vi "Initialize RF Sessions From Pinmap.vi"(0 "TSM Context":T1, 11 "error in":errorcluster) -> (4 "RF SubSystem Session Providers":refnum<class "RF Subsystem Session Provider.lvclass">[](array[class]), 15 "error out":errorcluster)   [LabVIEW 2023, in "RFFixtureCharact.Public.lvlib"]
uses:
  RFFixtureCharact.Public.lvlib
  <vilib>/NI_TestStand_SemiconductorModule/NI_TestStand_Semiconductor_Module.lvlibp/PinMap/General/SemiconductorModuleContext.ctl
  Common/RF Subsystem Session Provider/RF Subsystem Session Provider.lvclass
  Common/RFCalAndFixtureCharact.Common.lvlib
  <vilib>/NI_TestStand_SemiconductorModule/NI_TestStand_Semiconductor_Module.lvlibp
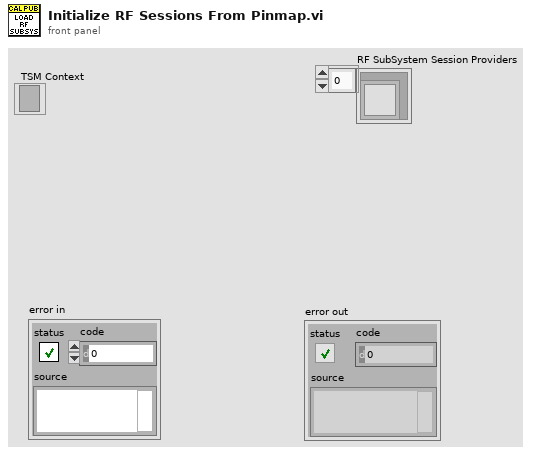
[diagram p1: front panel]
types:
  T1 = typedef "NI_TestStand_Semiconductor_Module.lvlibp/SemiconductorModuleContext.ctl" = refnum<k7>
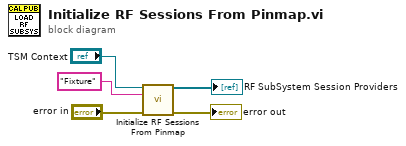
[diagram p0: block diagram]
diagram:
  n1 = call "Initialize RF Sessions From Pinmap.vi"("TSM Context"="TSM Context", "Fixture Or Cal"="Fixture", "Error in"="error in") -> ("RF SubSystem Session Providers"=→"RF SubSystem Session Providers":refnum<class "RF Subsystem Session Provider.lvclass">[], "Error out"=→"error out":errorcluster)  [unwired: 11 in]
